vi "Initialize with Topology (Simulate).vi"(8 "error in (no error)":errorcluster, 10 "topology":string, 11 "switches json":string) -> (0 "error out":errorcluster, 3 "session out":T1)   [LabVIEW 2020, in "SLSC Switch.lvlib"]
doc: "Returns a session handle used to identify the SLSC module in all subsequent SLSC Switch driver calls and sets the topology of the switch module."
uses:
  <vilib>/SLSC_Switch/SLSC Switch.lvlib
  nislscsl.dll
  <vilib>/userdefined/High Color/SLSC_Switch/nislscslSession.ctl
panel:
  in  "session in":T1
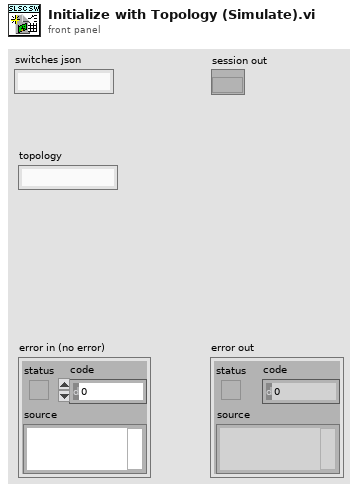
[diagram p1: front panel]
types:
  T1 = typedef "nislscslSession.ctl" = refnum<k20>
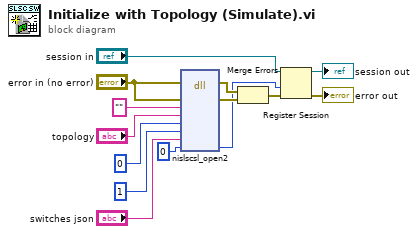
[diagram p0: block diagram]
diagram:
  n1 = dll-call lib="nislscsl.*" fn="nislscsl_open2"(error in="error in (no error)", "errorCluster"="error in (no error)", "deviceIdentifier"="", "topologyName"="topology", "reset"=u8 0, "simulate"=u8 1, "capabilities"="switches json", "sessionHandlePtr"=u64 0) -> (error out=w8:errorcluster, "errorCluster"=w9:errorcluster, "sessionHandlePtr"=w7:u64)  [unwired: 8 in, 1 out]
  n2 = Merge Errors(w8, w9) -> (w14:errorcluster)
  n3 = Register Session(8:w14, 9:w7, 11:"session in") -> (0:→"error out":errorcluster, 3:→"session out":T1)  [unwired: 2 in]
